vi "oa_Back Extrapolation Processing.vi"(9 "pulse history in [s]":dbl[](array[numeric]) format="%.2f", 10 "pulse new history in [s]":dbl[](array[numeric]) format="%.2f", 11 "pulse positions in [s]":dbl[](array[numeric]) format="%.2f") -> (0 "pulse future [s]":dbl[](array[numeric]) format="%.2f", 1 "pulse history out [s]":dbl[](array[numeric]) format="%.2f", 2 "pulse new history out [s]":dbl[](array[numeric]) format="%.2f", 3 "pulse positions out [s]":dbl[](array[numeric]) format="%.2f")   [LabVIEW 2017, in "SoundVib_TachProcess.lvlib"]
uses:
  <vilib>/addons/Sound and Vibration/Order Analysis/Tach Process/SoundVib_TachProcess.lvlib
  <vilib>/Analysis/NI_AALPro.lvlib
  <vilib>/Analysis/NI_AALBase.lvlib
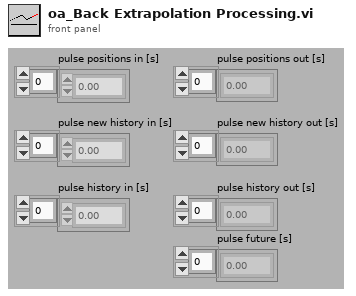
[diagram p1: front panel]
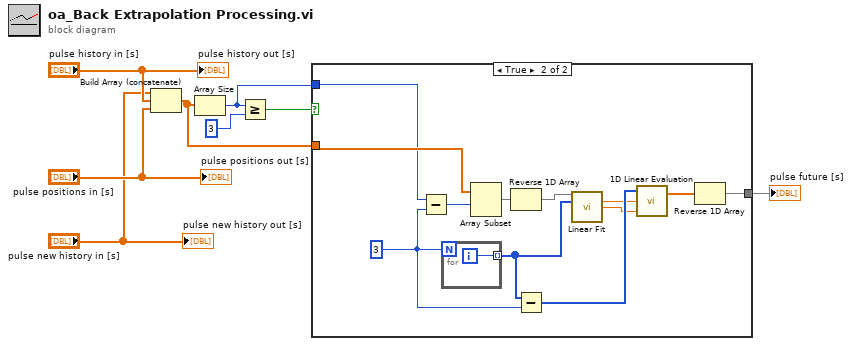
[diagram p0: block diagram]
diagram:
  n1 = Build Array (concatenate)("pulse new history in [s]", "pulse history in [s]", "pulse positions in [s]") -> (w7:dbl[])
  n2 = Array Size(array=w7) -> (size(s)=w2:i32)
  n3 = Greater Or Equal?(x=w2, y=3) -> (x >= y?=w6:bool)
  n4 = case shown="True" w6 {
    tunnel: w7 -> [_ w14]
    tunnel: [_ w11] -> w5
    tunnel: w2 -> [_ w9]
    frame False {
    }
    frame True {
      w15 = 3 ("extrapolation length")
      n5 = Subtract(x=w9, y=w15) -> (x-y=w20:i32)
      n6 = for {
        N: w15 -> [_]
        tunnel: [w21] -> w10 mode=indexing
        i -> [w21]
      }
      n7 = Array Subset(array=w14, index=w20) -> (w19:dbl[])  [unwired: 1 in]
      n8 = Reverse 1D Array(array=w19) -> (reversed array=w18:dbl[])
      n9 = Subtract(x=w10, y=w15) -> (x-y=w16:i32[])
      n10 = call <vilib>:"Linear Fit.vi"("Y"=w18, "X"=w10) -> ("slope"=w13:dbl, "intercept"=w12:dbl)  [unwired: 9 in, 3 out]
      n11 = call <vilib>:"1D Linear Evaluation.vi"("offset"=w12, "scale"=w13, "X"=w16) -> ("Y[i]=X[i]*a+b"=w17:dbl[])  [unwired: 1 out]
      n12 = Reverse 1D Array(array=w17) -> (reversed array=w11:dbl[])
    }
  }
  "pulse future [s]" <- w5
  "pulse positions out [s]" <- "pulse positions in [s]"
  "pulse history out [s]" <- "pulse history in [s]"
  "pulse new history out [s]" <- "pulse new history in [s]"
